vi "AD5781Init.vi"(8 "error in":errorcluster, 10 "SPI - AD5781 Setup":T2={"Port"=0, "Configuration Cluster"={"CS"=1, "Clock Rate (Hz)"=50000.0, "Clock Mode"=2, "CS Active State"=FALSE}, "Hardware Pins"={"RESET"=TRUE, "LDAC"=FALSE, "CLR"=TRUE}, "Total Bits"=8} {"Configuration Cluster"."CS" items=["0"=1, "1"=2, "2"=4, "3"=8, "4"=16, "5"=32, "6"=64, "7"=128]; "Configuration Cluster"."Clock Mode" items=["0", "1", "2", "3"]}, 11 "FPGA Interface":T3) -> (0 "error out":errorcluster, 2 "Read Data":u8[](array[numeric]) format="%08b", 3 "FPGA Interface 2":T3)   [LabVIEW 2014]
uses:
  Host API/Controls/FPGA Reference.ctl
  Host API/Controls/SPI Configuration Cluster.ctl
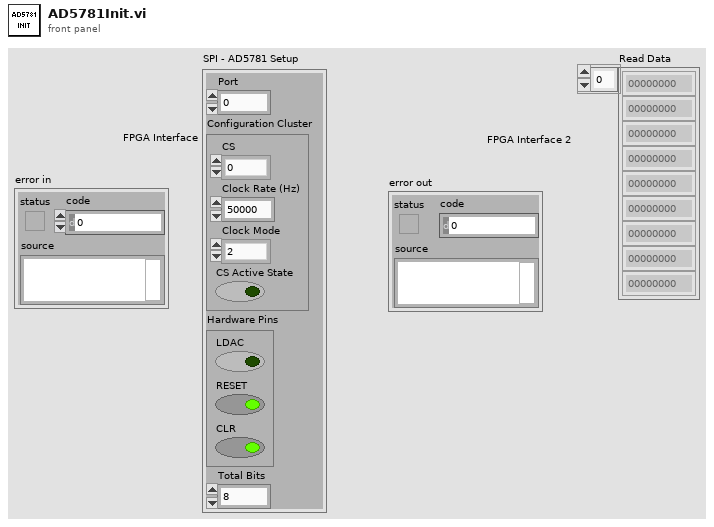
[diagram p1: front panel]
types:
  T1 = typedef "SPI Configuration Cluster.ctl" = cluster{"CS":u8, "Clock Rate (Hz)":dbl, "Clock Mode":u8, "CS Active State":bool}
  T2 = cluster{"Port":i8, "Configuration Cluster":T1, "Hardware Pins":cluster{"RESET":bool, "LDAC":bool, "CLR":bool}, "Total Bits":u16}
  T3 = typedef "FPGA Reference.ctl" = refnum<k20>
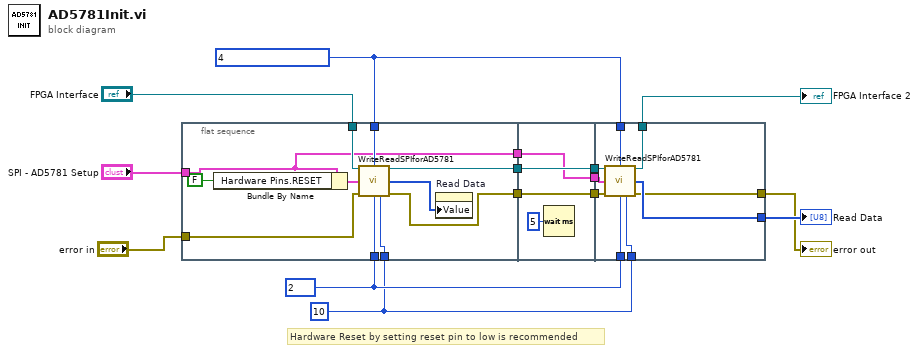
[diagram p0: block diagram]
diagram:
  w8 = u8 10 ("2-Bit Suffix")
  w9 = u8 2 ("register prefix")
  w7 = u32 4 ("Write Data")
  # "Hardware Reset by setting reset pin to low is recommended"
  n1 = flat-sequence {
    tunnel: "SPI - AD5781 Setup" -> [w17]
    tunnel: "error in" -> [w24]
    tunnel: "FPGA Interface" -> [w23]
    tunnel: [w22] -> w11
    tunnel: w9 -> [w20]
    tunnel: w8 -> [w19]
    tunnel: w7 -> [w18]
    tunnel: [w17] -> w6
    tunnel: [w16] -> w4
    tunnel: [w29] -> w12
    tunnel: w11 -> [w29]
    tunnel: w6 -> [w28]
    tunnel: [w28] -> w5
    tunnel: w4 -> [w27]
    tunnel: [w27] -> w3
    tunnel: w12 -> [w39]
    tunnel: [w38] -> w10
    tunnel: w9 -> [w37]
    tunnel: w8 -> [w36]
    tunnel: w7 -> [w35]
    tunnel: w5 -> [w34]
    tunnel: w3 -> [w33]
    tunnel: [w32] -> w2
    tunnel: [w31] -> w1
    frame #0 {
      n2 = Bundle By Name(cluster=w17, "Hardware Pins.RESET"=FALSE) -> (w25:T2)
      n3 = call "WriteReadSPIforAD5781.vi"("FPGA VI Reference Out 2"=w23, "DAC 18Bit Data"=w18, "SPI - AD5781 Setup"=w25, "error in"=w24, "register prefix"=w20, "2-Bit Suffix"=w19) -> ("FPGA VI Reference Out"=w22:T3, "Read Data"=w21:u8[], "error out"=w16:errorcluster)  [unwired: 7 in]
      n4 = property on="Read Data" class="Arr (strict)"("Value"=w21) -> ()  [unwired: 2 in, 2 out]
    }
    frame #1 {
      n5 = Wait (ms)(milliseconds to wait=u32 5) -> ()  [unwired: 1 out]
    }
    frame #2 {
      n6 = call "WriteReadSPIforAD5781.vi"("FPGA VI Reference Out 2"=w39, "DAC 18Bit Data"=w35, "SPI - AD5781 Setup"=w34, "error in"=w33, "register prefix"=w37, "2-Bit Suffix"=w36) -> ("FPGA VI Reference Out"=w31:T3, "Read Data"=w38:u8[], "error out"=w32:errorcluster)  [unwired: 7 in]
    }
  }
  "FPGA Interface 2" <- w1
  "error out" <- w2
  "Read Data" <- w10
